vi "UserVars-Expression PDF.vi"(0 "Expr":string, 11 "error in (no error)":errorcluster) -> (4 "X":dbl[](array[numeric]), 6 "PDF":dbl[](array[numeric]), 8 "refpts":dbl[](array[numeric]), 10 "mass function":bool, 15 "error out":errorcluster)   [LabVIEW 2020]
uses:
  <vilib>/Analysis/baseanly.llb/Mean (DBL).vi
  <vilib>/gmath/NI_Gmath.lvlib
  <vilib>/Analysis/NI_AALBase.lvlib
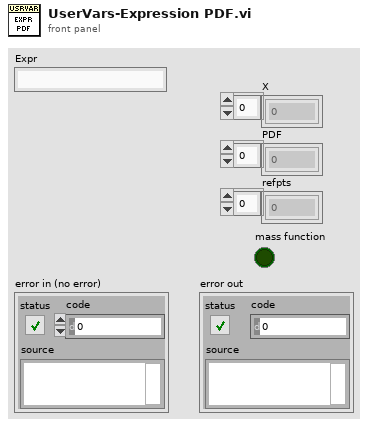
[diagram p1: front panel]
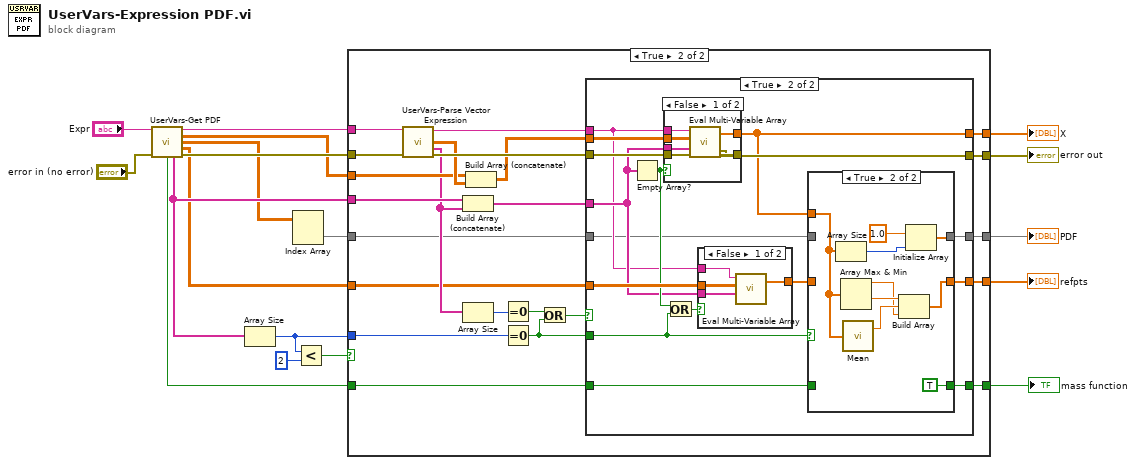
[diagram p0: block diagram]
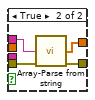
[diagram p6: hidden frame]
diagram:
  n1 = call "UserVars-Get PDF.vi"("Expr in"="Expr", "error in (no error)"="error in (no error)") -> ("Expr out"=w17:string, "X"=w15:dbl[][], "PDF"=w6:dbl[][], "Ref Pts"=w8:dbl[][], "mass function"=w9:bool, "Vars"=w12:string[], "error out"=w16:errorcluster)  [unwired: 7 in]
  n2 = Array Size(array=w12) -> (size(s)=w11:i32)
  n3 = Index Array(array=w6) -> (element=w5:dbl[])  [unwired: 2 in]
  n4 = Less?(x=w11, y=2) -> (x < y?=w13:bool)
  n5 = case shown="True" w13 {
    tunnel: [w19 w42] -> w18
    tunnel: w17 -> [_ w41]
    tunnel: w16 -> [w19 w40]
    tunnel: w12 -> [_ w36]
    tunnel: [_ w33] -> w10
    tunnel: w15 -> [_ w32]
    tunnel: w11 -> [_ w29]
    tunnel: w9 -> [_ w21]
    tunnel: w8 -> [_ w25]
    tunnel: [_ w24] -> w7
    tunnel: w5 -> [_ w23]
    tunnel: [_ w22] -> w4
    tunnel: [_ w20] -> w3
    frame False {
    }
    frame True {
      n6 = call "UserVars-Parse Vector Expression.vi"("Expression In"=w41, "error in (no error)"=w40) -> ("Expression Out"=w38:string, "values"=w37:dbl[][], "variables"=w31:string[], "error out"=w39:errorcluster)  [unwired: 10 in]
      n7 = Build Array (concatenate)(w36, w31) -> (w35:string[])
      n8 = Array Size(array=w31) -> (size(s)=w30:i32)
      n9 = Build Array (concatenate)(w32, w37) -> (w34:dbl[][])
      n10 = Equal To 0?(x=w30) -> (x = 0?=w28:bool)
      n11 = Equal To 0?(x=w29) -> (x = 0?=w26:bool)
      n12 = Or(x=w28, y=w26) -> (x .or. y?=w27:bool)
      n13 = case shown="True" w27 {
        tunnel: [w43 w59] -> w42
        tunnel: w39 -> [w43 w58]
        tunnel: w38 -> [_ w52]
        tunnel: w35 -> [_ w53]
        tunnel: w34 -> [_ w57]
        tunnel: [_ w44] -> w33
        tunnel: w26 -> [_ w51]
        tunnel: w25 -> [_ w56]
        tunnel: [_ w49] -> w24
        tunnel: w23 -> [_ w50]
        tunnel: [_ w47] -> w22
        tunnel: w21 -> [_ w46]
        tunnel: [_ w45] -> w20
        frame False {
        }
        frame True {
          n14 = Empty Array?(array=w53) -> (empty?=w55:bool)
          n15 = case shown="False" w55 {
            tunnel: w52 -> [w81 w84]
            tunnel: w57 -> [w80 _]
            tunnel: w53 -> [w79 _]
            tunnel: w58 -> [w78 w82]
            tunnel: [w77 w85] -> w59
            tunnel: [w76 w83] -> w44
            frame False {
              n16 = call <vilib>:"Eval Multi-Variable Array.vi"("error in (no error)"=w78, "Variables"=w79, "X Values"=w80, "formula"=w81) -> ("error out"=w77:errorcluster, "Y Values"=w76:dbl[])
            }
            frame True {
              n17 = call "Array-Parse from string.vi"("String"=w84, "error in (no error)"=w82) -> ("Array"=w83:dbl[], "error out"=w85:errorcluster)  [unwired: 12 in]
            }
          }
          n18 = Or(x=w55, y=w51) -> (x .or. y?=w54:bool)
          n19 = case shown="False" w54 {
            tunnel: w56 -> [w75 _]
            tunnel: w53 -> [w74 _]
            tunnel: w52 -> [w73 _]
            tunnel: [w72 _] -> w48
            frame False {
              n20 = call <vilib>:"Eval Multi-Variable Array.vi"("Variables"=w74, "X Values"=w75, "formula"=w73) -> ("Y Values"=w72:dbl[])  [unwired: 1 in, 1 out]
            }
            frame True {
            }
          }
          n21 = case shown="True" w51 {
            tunnel: w50 -> [w61 _]
            tunnel: [w62 w64] -> w49
            tunnel: w48 -> [w62 _]
            tunnel: [w61 w71] -> w47
            tunnel: w46 -> [w60 _]
            tunnel: [w60 TRUE ("mass function")] -> w45
            tunnel: w44 -> [_ w68]
            frame False {
            }
            frame True {
              n22 = Array Size(array=w68) -> (size(s)=w69:i32)
              n23 = Array Max & Min(array=w68) -> (max value=w65:dbl, min value=w67:dbl)  [unwired: 2 out]
              n24 = call-poly <vilib>:"Mean.vi"("X"=w68) -> ("mean"=w66:dbl)  [unwired: 1 out]
              n25 = Build Array(w67, w66, w65) -> (w64:dbl[])
              n26 = Initialize Array(1.0, w69) -> (w71:dbl[])
            }
          }
        }
      }
    }
  }
  "error out" <- w18
  "X" <- w10
  "PDF" <- w4
  "refpts" <- w7
  "mass function" <- w3
